vi "tc_selection.vi"(10 "Coords":T1, 11 "Position":T2) -> (3 "Boolean":bool)   [LabVIEW 2017]
uses:
  <vilib>/Utility/miscctls.llb/LVPositionTypeDef.ctl
  <vilib>/Utility/miscctls.llb/LVPoint32TypeDef.ctl
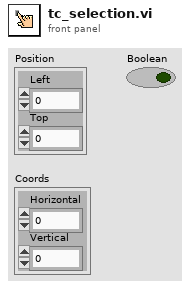
[diagram p1: front panel]
types:
  T1 = typedef "LVPoint32TypeDef.ctl" = cluster{"Horizontal":i32, "Vertical":i32}
  T2 = typedef "LVPositionTypeDef.ctl" = cluster{"Left":i32, "Top":i32}
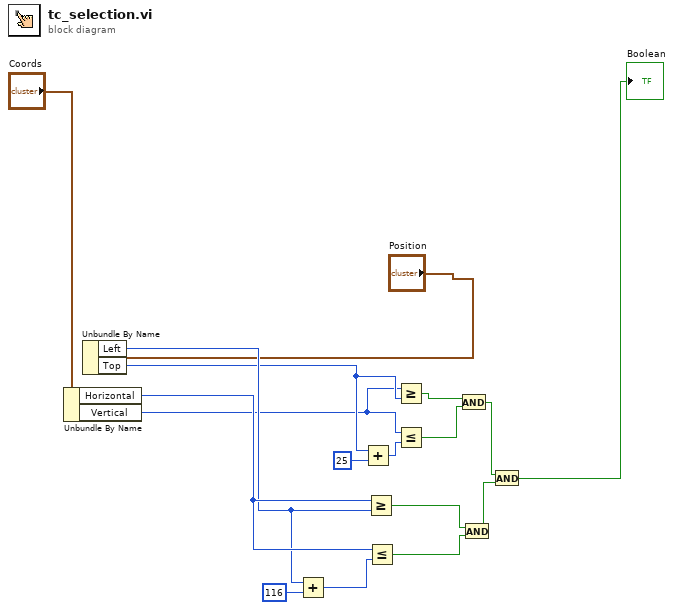
[diagram p0: block diagram]
diagram:
  n1 = Unbundle By Name("Coords") -> ("Horizontal"=w13:i32, "Vertical"=w7:i32)
  n2 = Unbundle By Name("Position") -> ("Left"=w10:i32, "Top"=w8:i32)
  n3 = Add(x=w10, y=116) -> (x+y=w11:i32)
  n4 = Add(x=w8, y=25) -> (x+y=w6:i32)
  n5 = Greater Or Equal?(x=w13, y=w10) -> (x >= y?=w9:bool)
  n6 = Less Or Equal?(x=w13, y=w11) -> (x <= y?=w14:bool)
  n7 = Greater Or Equal?(x=w7, y=w8) -> (x >= y?=w3:bool)
  n8 = Less Or Equal?(x=w7, y=w6) -> (x <= y?=w4:bool)
  n9 = And(x=w3, y=w4) -> (x .and. y?=w16:bool)
  n10 = And(x=w9, y=w14) -> (x .and. y?=w15:bool)
  n11 = And(x=w16, y=w15) -> (x .and. y?=→"Boolean":bool)
